vi "UAXMLParse.vi"(8 "error in (no error)":errorcluster caption="错误输入（无错误）", 10 "label":string="opcua_server", 11 "string":string="<opcua_server><name>server</name><port>4845</port><policy>none</policy><serverCertification></serverCertification><trustedClientCertifications><certification></certification></trustedClientCertifications><structure><folder name=\"all supported datatypes\"><folder name=\"singal element\"><item name=\"boolean\" access=\"read/write\" datatype=\"boolean\" initialValue=\"TRUE\"></item><item name=\"string\" access=\"read/write\" datatype=\"string\" initialValue=\"stringtype\"></item><item name=\"sbyte\" access=\"read/write\" datatype=\"sbyte\" initialValue=\"-10\"></item><item name=\"byte\" access=\"read/write\" datatype=\"byte\" initialValue=\"10\"></item><item name=\"int16\" access=\"read/write\" datatype=\"int16\" initialValue=\"-10\"></item><item name=\"int32\" access=\"read/write\" datatype=\"int32\" initialValue=\"-20\"></item><item name=\"int64\" access=\"read/write\" datatype=\"int64\" initialValue=\"-30\"></item><item name=\"uint16\" access=\"read/write\" datatype=\"uint16\" initialValue=\"10\"></item><item name=\"uint32\" access=\"read/write\" datatype=\"uint32\" initialValue=\"20\"></item><item name=\"uint64\" access=\"read/write\" datatype=\"uint64\" initialValue=\"30\"></item><item name=\"double\" access=\"read/write\" datatype=\"double\" initialValue=\"10.1\"></item><item name=\"float\" access=\"read/write\" datatype=\"float\" initialValue=\"12.1\"></item><item name=\"datetime\" access=\"read/write\" datatype=\"datetime\" initialValue=\"4/30/2004 7:48:47 PM\"></item><item name=\"byte string\" access=\"read/write\" datatype=\"ByteString\" initialValue=\"(1,2,3,4,5)\"></item></folder><folder name=\"array\"><item name=\"boolean array\" access=\"read/write\" datatype=\"boolean array\" initialValue=\"FALSE,TRUE,FALSE\"></item><item name=\"string array\" access=\"read/write\" datatype=\"string array\" initialValue=\"str1,str2,str3\"></item><item name=\"sbyte array\" access=\"read/write\" datatype=\"sbyte array\" initialValue=\"-1,2,-3,4,-5,6,-7,8\"></item><item name=\"byte array\" access=\"read/write\" datatype=\"byte array\" initialValue=\"1,2,3,4,5,6,7,8\"></item><item name=\"int16 array\" access=\"read/write\" datatype=\"int16 array\" initialValue=\"-1,2,-3,4,-5,6,-7,8\"></item><item name=\"int32 array\" access=\"read/write\" datatype=\"int32 array\" initialValue=\"-1,2,-3,4,-5,6,-7,8\"></item><item name=\"int64 array\" access=\"read/write\" datatype=\"int64 array\" initialValue=\"-1,2,-3,4,-5,6,-7,8\"></item><item name=\"uint16 array\" access=\"read/write\" datatype=\"uint16 array\" initialValue=\"1,2,3,4,5,6,7,8\"></item><item name=\"uint32 array\" access=\"read/write\" datatype=\"uint32 array\" initialValue=\"1,2,3,4,5,6,7,8\"></item><item name=\"uint64 array\" access=\"read/write\" datatype=\"uint64 array\" initialValue=\"1,2,3,4,5,6,7,8\"></item><item name=\"double array\" access=\"read/write\" datatype=\"double array\" initialValue=\"1.1,2.2,3.3\"></item><item name=\"float array\" access=\"read/write\" datatype=\"float array\" initialValue=\"1.1,2.2,3.3\"></item><item name=\"datetime array\" access=\"read/write\" datatype=\"datetime array\" initialValue=\"4/30/2004 7:48:47 PM,5/30/2004 8:48:47 PM,6/30/2004 9:48:47 PM\"></item></folder></folder><folder name=\"structure demo\"><folder name=\"device1\"><item name=\"int1\" access=\"read/write\" datatype=\"int32\" initialValue=\"50\" description=\"\"><property name=\"set point\" access=\"read/write\" datatype=\"int32\" initialValue=\"12.4\" description=\"Set point of int1.\"></property><property name=\"status\" access=\"read only\" datatype=\"boolean\" initialValue=\"FALSE\" description=\"Status of int1.\"></property></item></folder><folder name=\"device2\"><folder name=\"device3\"><item name=\"bool1\" access=\"read/write\" datatype=\"boolean\" initialValue=\"FALSE\" description=\"\"><property name=\"set point\" access=\"read/write\" datatype=\"boolean\" initialValue=\"FALSE\" description=\"Set point of bool1.\"></property><property name=\"status\" access=\"read only\" datatype=\"boolean\" initialValue=\"FALSE\" description=\"Status of bool1.\"></property></item></folder><item name=\"str1\" access=\"read/write\" datatype=\"string\" initialValue=\"\" description=\"\"><property name=\"set point\" access=\"read/write\" datatype=\"string\" initialValue=\"test initialize\" description=\"Set point of str1.\"></property><property name=\"status\" access=\"read only\" datatype=\"boolean\" initialValue=\"FALSE\" description=\"Status of str1.\"></property></item></folder><folder name=\"grandpa\"><folder name=\"father\"><folder name=\"son\"><item name=\"son item\" access=\"read/write\" datatype=\"string\" initialValue=\"\" description=\"\"></item></folder></folder></folder><folder name=\"level1\"><folder name=\"level2\"><folder name=\"level3\"><folder name=\"level4\"><folder name=\"level5\"><folder name=\"level6\"><item name=\"data level6\" access=\"read/write\" datatype=\"uint32\" initialValue=\"1000\" description=\"\"></item></folder></folder></folder></folder></folder></folder></folder></structure></opcua_server>") -> (0 "error out":errorcluster caption="错误输出", 1 "keyValues":cluster{"key":string, "value":string}[](array[cluster]), 2 "match substring":string, 3 "content":string, 5 "after substring":string, 7 "before substring":string)   [LabVIEW 2014, in "OPCUA XML(dev).lvlib"]
uses:
  OPCUA XML(dev).lvlib
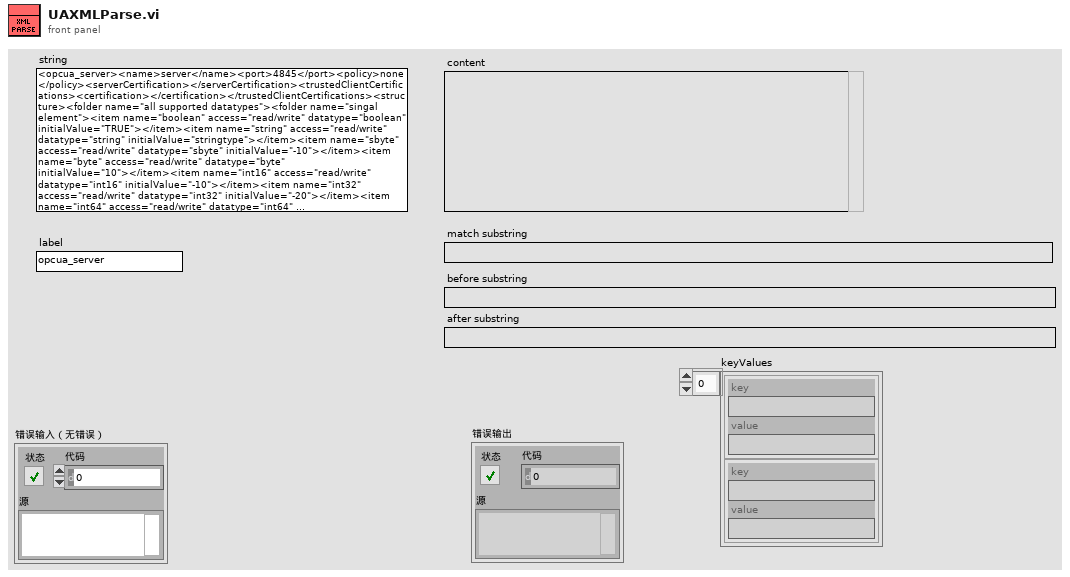
[diagram p1: front panel]
types:
  T1 = cluster{"whole match":string, "whole match":string}[]
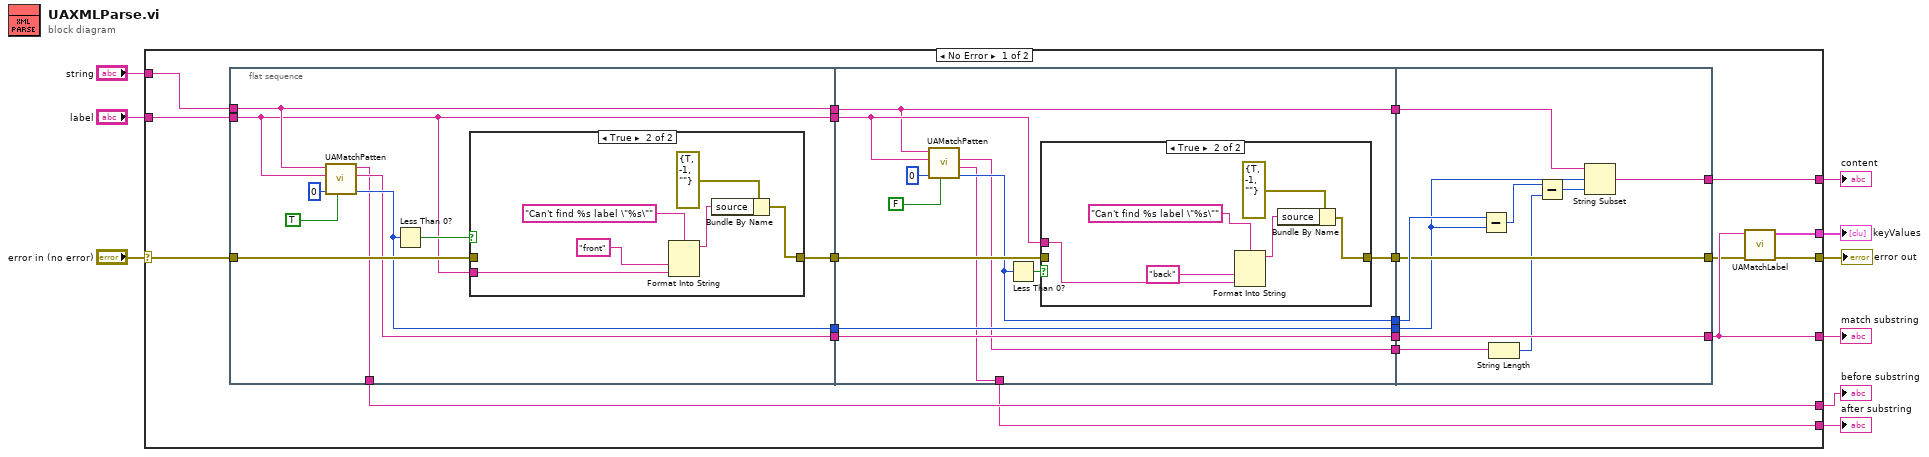
[diagram p0: block diagram]
diagram:
  n1 = case shown="No Error" "error in (no error)" {
    selector: "error in (no error)" -> [w28 w77]
    tunnel: [w11 w77] -> w8
    tunnel: "label" -> [w29 _]
    tunnel: "string" -> [w30 _]
    tunnel: [w17 _] -> w5
    tunnel: [w16 _] -> w4
    tunnel: [w15 _] -> w3
    tunnel: [w13 _] -> w2
    tunnel: [w10 _] -> w1
    frame No Error {
      n2 = flat-sequence {
        tunnel: w30 -> [w36]
        tunnel: w29 -> [w31]
        tunnel: w28 -> [w38]
        tunnel: [w37] -> w27
        tunnel: [w31] -> w26
        tunnel: [w36] -> w25
        tunnel: [w35] -> w22
        tunnel: [w34] -> w20
        tunnel: [w32] -> w16
        tunnel: w27 -> [w57]
        tunnel: w26 -> [w51]
        tunnel: w25 -> [w48]
        tunnel: [w48] -> w24
        tunnel: [w56] -> w23
        tunnel: w22 -> [w56]
        tunnel: [w55] -> w21
        tunnel: w20 -> [w54]
        tunnel: [w54] -> w19
        tunnel: [w53] -> w18
        tunnel: [w50] -> w15
        tunnel: [w49] -> w14
        tunnel: w24 -> [w76]
        tunnel: w23 -> [w71]
        tunnel: w21 -> [w75]
        tunnel: w19 -> [w72]
        tunnel: [w74] -> w12
        tunnel: w18 -> [w74]
        tunnel: [w73] -> w17
        tunnel: [w72] -> w13
        tunnel: w14 -> [w69]
        frame #0 {
          n3 = call "UAMatchPatten.vi"("first(T)/Last(F)"=TRUE, "offset (0)"=0, "regular expression"=w31, "string"=w36) -> ("offset past match"=w35:i32, "concatenated string out"=w34:string, "before substring"=w32:string)  [unwired: 4 in, 1 out]
          n4 = Less Than 0?(x=w35) -> (x < 0?=w39:bool)
          n5 = case shown="True" w39 {
            tunnel: w38 -> [w41 _]
            tunnel: [w41 w46] -> w37
            tunnel: w31 -> [_ w43]
            frame False {
            }
            frame True {
              n6 = Format Into String(format string="Can't find %s label \"%s\"", "front" ("format string"), w43) -> (resulting string=w45:string)  [unwired: 2 in, 1 out]
              n7 = Bundle By Name(cluster=errorcluster {"status"=TRUE, "code"=-1, "source"=""} ("error IO"), "source"=w45) -> (w46:errorcluster)
            }
          }
        }
        frame #1 {
          n8 = call "UAMatchPatten.vi"("first(T)/Last(F)"=FALSE, "offset (0)"=0, "regular expression"=w51, "string"=w48) -> ("offset past match"=w55:i32, "after substring"=w50:string, "concatenated string out"=w49:string)  [unwired: 4 in, 1 out]
          n9 = Less Than 0?(x=w55) -> (x < 0?=w58:bool)
          n10 = case shown="True" w58 {
            tunnel: [w60 w65] -> w53
            tunnel: w51 -> [_ w62]
            tunnel: w57 -> [w60 _]
            frame False {
            }
            frame True {
              n11 = Format Into String(format string="Can't find %s label \"%s\"", "back" ("format string"), w62) -> (resulting string=w64:string)  [unwired: 2 in, 1 out]
              n12 = Bundle By Name(cluster=errorcluster {"status"=TRUE, "code"=-1, "source"=""} ("error IO"), "source"=w64) -> (w65:errorcluster)
            }
          }
        }
        frame #2 {
          n13 = Subtract(x=w75, y=w71) -> (x-y=w68:i32)
          n14 = String Length(string=w69) -> (length=w70:i32)
          n15 = Subtract(x=w68, y=w70) -> (x-y=w67:i32)
          n16 = String Subset(string=w76, offset (0)=w71, length (rest)=w67) -> (substring=w73:string)
        }
      }
      n17 = call "UAMatchLabel.vi"("error in (no error)"=w12, "String"=w13) -> ("error out"=w11:errorcluster, "keyValues"=w10:T1)  [unwired: 8 in]
    }
    frame Error {
    }
  }
  "error out" <- w8
  "content" <- w5
  "match substring" <- w2
  "after substring" <- w3
  "before substring" <- w4
  "keyValues" <- w1
